vi "Transfer to DMA.vi"(8 "error in (no error)":errorcluster, 9 "Transfer in":refnum<class "Transfer.lvclass">, 10 "DMA Transfer Spec in":T1 {"Block Descriptors"."descriptor params"."data ptr (lower)" format="%.0x"; "Block Descriptors"."descriptor params"."data ptr (upper)" format="%.0x"; "Block Descriptors"."descriptor params"."data size" format="%.0x"; "Block Descriptors"."descriptor params"."next descriptor ptr" format="%.0x"; "Block Descriptors"."descriptor size" format="%08x"; "Block Descriptors"."descriptor ptr (RFM)" format="%08x"; "Block Descriptors"."descriptor ptr (VISA)" format="%08x"; "RFM offset" format="%08x"}, 11 "GE 5565PIORC in":refnum<class "GE 5565PIORC.lvclass">) -> (0 "error out":errorcluster, 1 "Transfer out":refnum<class "Transfer.lvclass">, 2 "DMA Transfer Spec out":T1 {"Block Descriptors"."descriptor params"."data ptr (lower)" format="%.0x"; "Block Descriptors"."descriptor params"."data ptr (upper)" format="%.0x"; "Block Descriptors"."descriptor params"."data size" format="%.0x"; "Block Descriptors"."descriptor params"."next descriptor ptr" format="%.0x"; "Block Descriptors"."descriptor size" format="%08x"; "Block Descriptors"."descriptor ptr (RFM)" format="%08x"; "Block Descriptors"."descriptor ptr (VISA)" format="%08x"; "RFM offset" format="%08x"}, 3 "GE 5565PIORC out":refnum<class "GE 5565PIORC.lvclass">)   [LabVIEW 2020, in "GE Reflective Memory.lvlib" / "GE Reflective Memory Transceiver.lvclass"]
uses:
  GE Reflective Memory Transceiver.lvclass
  Driver/Source/Typedefs/GE 5565PIORC.Typedef.DMA Transfer Spec.ctl
  Driver/Source/Typedefs/GE 5565PIORC.Typedef.DMA Block Descriptor.ctl
  Driver/Source/Typedefs/GE 5565PIORC.Typedef.DMA Block Descriptor Params.ctl
  DSF Core.lvlibp/Classes/Transfer/Transfer.lvclass
  Driver/Source/GE 5565PIORC.lvclass
  Driver/Source/GE 5565PIORC.lvclass/GE 5565PIORC.ctl
  Driver/Source/Methods/GE 5565PIORC.DMA.Get Transfer Components (Block).vi
  Driver/Source/Methods/GE 5565PIORC.DMA.Block.Write (String).vi
  Driver/Source/Properties/GE 5565PIORC.Read VISA MEMACC.vi
  DSF Core.lvlibp/Classes/Buffer/Buffer.lvclass
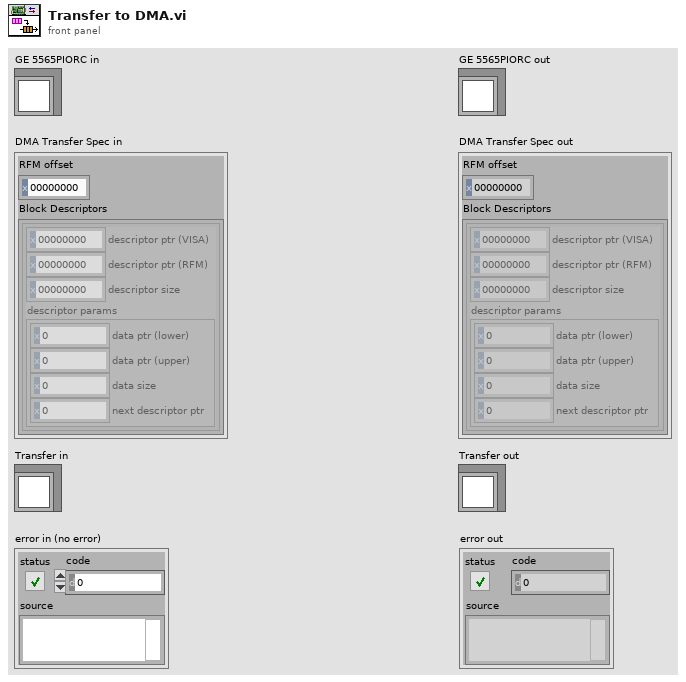
[diagram p1: front panel]
types:
  T1 = typedef "GE 5565PIORC.lvclass/GE 5565PIORC.Typedef.DMA Transfer Spec.ctl" = cluster{"RFM offset":u32, "Block Descriptors":T2[]}
  T2 = typedef "GE 5565PIORC.lvclass/GE 5565PIORC.Typedef.DMA Block Descriptor.ctl" = cluster{"descriptor ptr (VISA)":u32, "descriptor ptr (RFM)":u32, "descriptor size":u32, "descriptor params":T3}
  T3 = typedef "GE 5565PIORC.lvclass/GE 5565PIORC.Typedef.DMA Block Descriptor Params.ctl" = cluster{"data ptr (lower)":u32, "data ptr (upper)":u32, "data size":u32, "next descriptor ptr":u32}
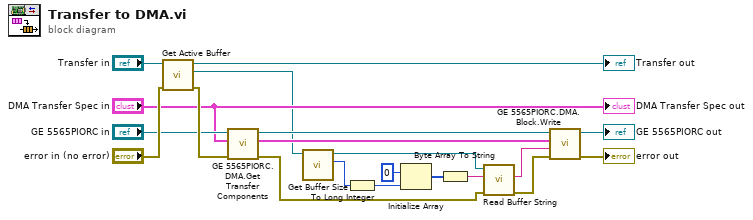
[diagram p0: block diagram]
diagram:
  n1 = call "Get Active Buffer.vi"("error in (no error)"="error in (no error)", "Transfer in"="Transfer in") -> ("error out"=w20:errorcluster, "Buffer"=w10:refnum<class "Buffer.lvclass">, "Transfer out"=→"Transfer out":refnum<class "Transfer.lvclass">)  [unwired: 7 in]
  n2 = call-poly "GE 5565PIORC.DMA.Get Transfer Components.vi"("error in (no error)"=w20, "DMA Transfer Spec in"="DMA Transfer Spec in", "GE 5565PIORC in"="GE 5565PIORC in") -> ("error out"=w2:errorcluster, "Block Descriptor"=w18:T2, "GE 5565PIORC out"=w17:refnum<class "GE 5565PIORC.lvclass">)  [unwired: 5 in, 1 out]
  n3 = call "Get Buffer Size.vi"("Buffer in"=w10) -> ("buffer size"=w9:u64, "Buffer out"=w4:refnum<class "Buffer.lvclass">)  [unwired: 9 in]
  n4 = To Long Integer(number=w9) -> (32bit integer=w8:i32)
  n5 = Initialize Array(u8 0 ("element"), w8) -> (w6:u8[])
  n6 = Byte Array To String(unsigned byte array=w6) -> (string=w5:string)
  n7 = call "Read Buffer String.vi"("error in (no error)"=w2, "dst string in"=w5, "Buffer in"=w4) -> ("error out"=w1:errorcluster, "dst string out"=w3:string)  [unwired: 5 in, 2 out]
  n8 = call-poly "GE 5565PIORC.DMA.Block.Write.vi"("error in (no error)"=w1, "data"=w3, "Block Descriptor in"=w18, "GE 5565PIORC in"=w17) -> ("error out"=→"error out":errorcluster, "GE 5565PIORC out"=→"GE 5565PIORC out":refnum<class "GE 5565PIORC.lvclass">)  [unwired: 4 in, 2 out]
  "DMA Transfer Spec out" <- "DMA Transfer Spec in"
